vi "Read TimeArray.vi"(8 "error in (no error)":errorcluster, 11 "EventPluginBaseClass in":refnum<class "EventPluginBaseClass.lvclass">) -> (0 "error out":errorcluster, 2 "dblTimeArray":dbl[](array[numeric]), 3 "EventPluginBaseClass out":refnum<class "EventPluginBaseClass.lvclass">)   [LabVIEW 2014, in "EventPlugins.lvlib" / "EventPluginBaseClass.lvclass"]
uses:
  EventPluginBaseClass.lvclass
  EventPluginBaseClass.lvclass/EventPluginBaseClass.ctl
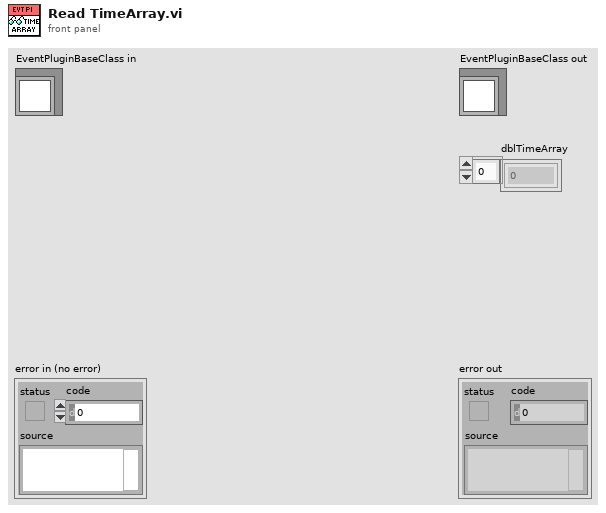
[diagram p1: front panel]
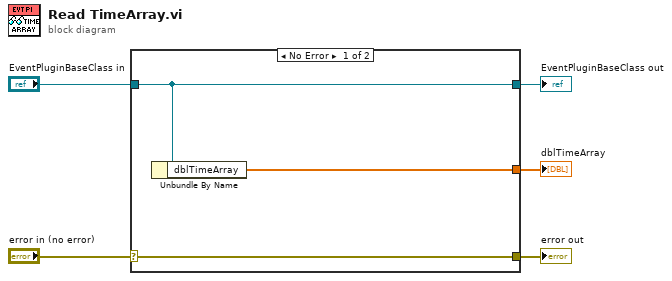
[diagram p0: block diagram]
diagram:
  n1 = case shown="No Error" "error in (no error)" {
    selector: "error in (no error)" -> [w8 w9]
    tunnel: [w8 w9] -> w4
    tunnel: [w7 w10] -> w2
    tunnel: "EventPluginBaseClass in" -> [w7 w10]
    tunnel: [w6 _] -> w1
    frame No Error {
      n2 = Unbundle By Name(w7) -> ("dblTimeArray"=w6:dbl[])
    }
    frame Error {
    }
  }
  "error out" <- w4
  "EventPluginBaseClass out" <- w2
  "dblTimeArray" <- w1
